vi "Wait_for_trigger_from_microscope.vi"   [LabVIEW 2016]
uses:
  Globals/LJ_Handles_Global.vi
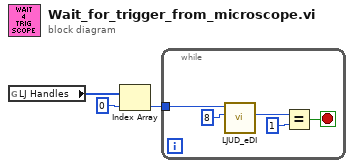
[diagram p0: block diagram]
diagram:
  n1 = global read "LJ_Handles_Global.vi" "LJ Handles"() -> (w2:i32[])
  n2 = Index Array(array=w2, index=0) -> (element=w1:i32)
  n3 = while {
    tunnel: w1 -> [w8]
    stop <- w4 stop-if-true
    n4 = call "LJUD_eDI.vi"("Channel"=8, "Handle In"=w8) -> ("State"=w6:i32)  [unwired: 7 in, 2 out]
    n5 = Equal?(x=w6, y=1) -> (x = y?=w4:bool)
  }
